vi "GetMfgDateCode.vi"(2 "error in (no error)":errorcluster, 3 "Delay Msecs (3000)":u32=3000, 4 "quit? (T)":bool=TRUE) -> (0 "error out":errorcluster, 1 "WeekYearCode":string)   [LabVIEW 2013]
panel:
  out "WeekYearCode for given":string
  in  "Time Stamp":timestamp
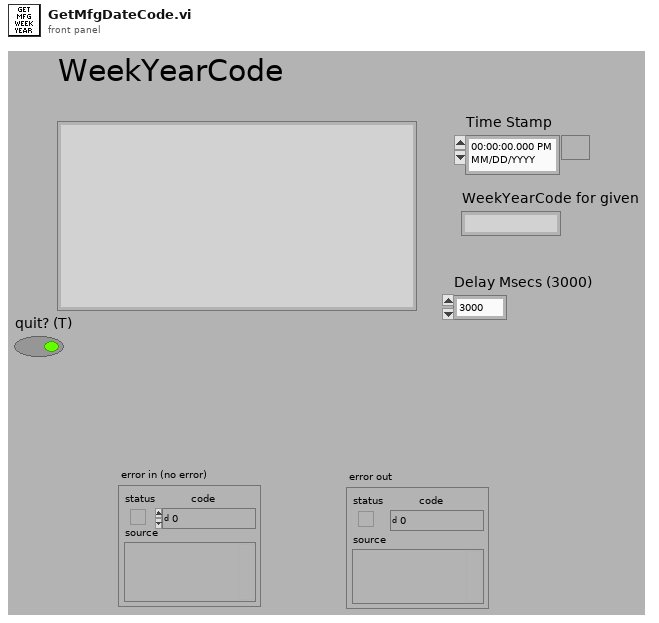
[diagram p1: front panel]
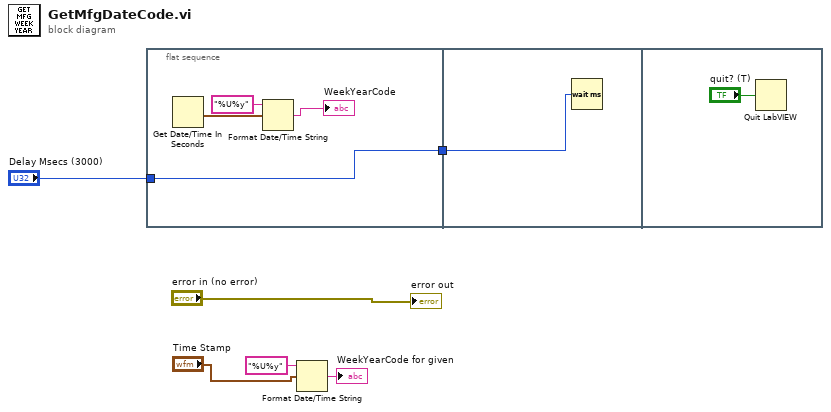
[diagram p0: block diagram]
diagram:
  n1 = flat-sequence {
    tunnel: [w7] -> w2
    tunnel: "Delay Msecs (3000)" -> [w7]
    tunnel: w2 -> [w11]
    frame #0 {
      n2 = Get Date/Time In Seconds() -> (seconds since 1Jan1904=w10:timestamp)
      n3 = Format Date/Time String(time format string (%c)="%U%y", seconds (now)=w10) -> (date/time string=→"WeekYearCode":string)  [unwired: 1 in]
    }
    frame #1 {
      n4 = Wait (ms)(milliseconds to wait=w11) -> ()  [unwired: 1 out]
    }
    frame #2 {
      n5 = Quit LabVIEW(quit? (T)="quit? (T)") -> ()
    }
  }
  n6 = Format Date/Time String(time format string (%c)="%U%y", seconds (now)="Time Stamp") -> (date/time string=→"WeekYearCode for given":string)  [unwired: 1 in]
  "error out" <- "error in (no error)"
